vi "GetChEnabled.vi"(0 "object in":refnum<class "AFG3022B_OJ.lvclass">, 5 "error in (no error)":errorcluster) -> (14 "object out":refnum<class "AFG3022B_OJ.lvclass">, 16 "Ch Enabled":cluster{"Ch1Enabled":bool, "Ch2Enabled":bool}, 19 "error out":errorcluster)   [LabVIEW 2023, in "AFG3022B_OJ.lvclass"]
uses:
  AFG3022B_OJ.lvclass
  AFG3022B_OJ.lvclass/AFG3022B_OJ.ctl
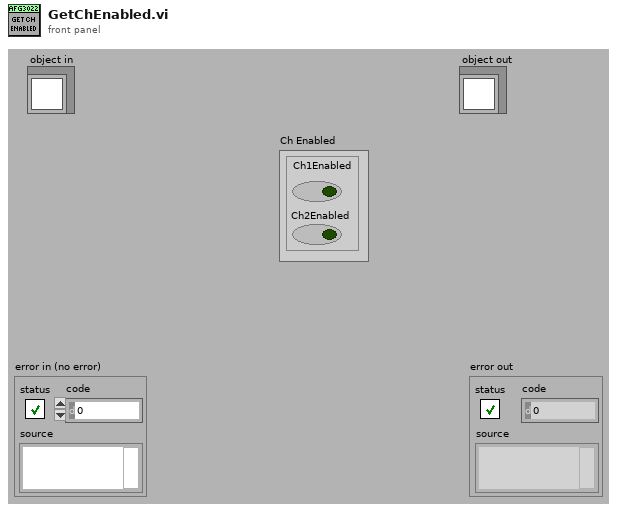
[diagram p1: front panel]
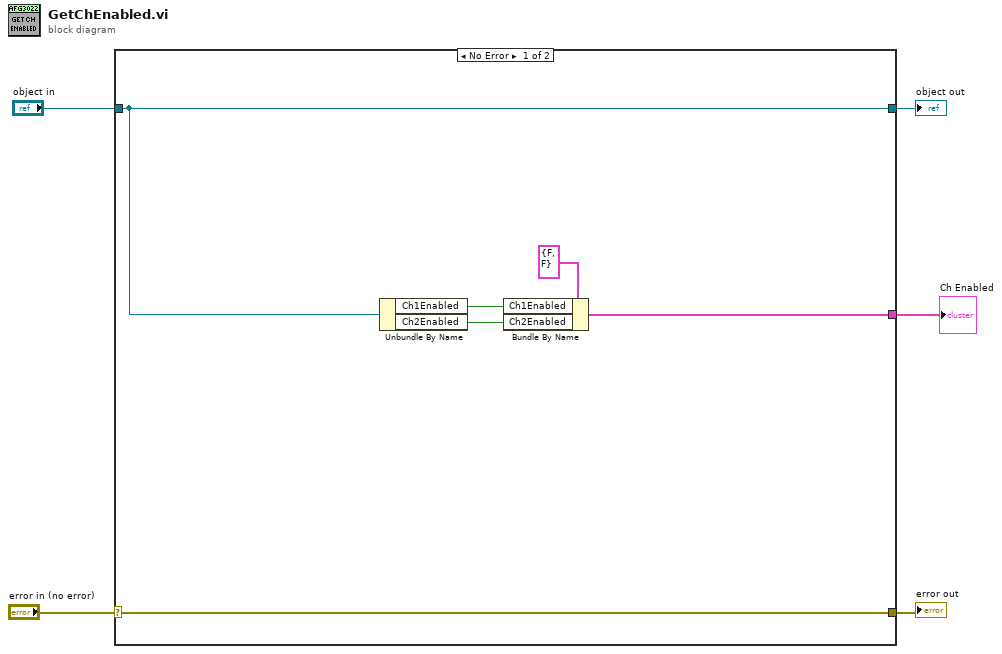
[diagram p0: block diagram]
diagram:
  n1 = case shown="No Error" "error in (no error)" {
    selector: "error in (no error)" -> [w11 w13]
    tunnel: [w11 w13] -> w4
    tunnel: [w10 w12] -> w2
    tunnel: "object in" -> [w10 w12]
    tunnel: [w6 _] -> w1
    frame No Error {
      n2 = Unbundle By Name(w10) -> ("Ch1Enabled"=w7:bool, "Ch2Enabled"=w8:bool)
      n3 = Bundle By Name(cluster=cluster{"Ch1Enabled":bool, "Ch2Enabled":bool} {"Ch1Enabled"=FALSE, "Ch2Enabled"=FALSE} ("Cluster"), "Ch1Enabled"=w7, "Ch2Enabled"=w8) -> (w6:cluster{"Ch1Enabled":bool, "Ch2Enabled":bool})
    }
    frame Error {
    }
  }
  "error out" <- w4
  "object out" <- w2
  "Ch Enabled" <- w1
